vi "Draw Button Background.vi"(6 "Button Color":u32(colorbox)=11776947, 8 "error in (no error)":errorcluster, 10 "Button Size":i32=40, 11 "Button Style":T1=enum."Classic") -> (0 "error out":errorcluster={"status"=TRUE, "code"=1131, "source"="Property Node (arg 1) in Toolbar.xctl:Draw Button Background.vi<APPEND>\nProperty Name: <b>Colors [4]</b>"}, 1 "On Picture":picture, 2 "Hover Picture":picture, 3 "Off Picture":picture)   [LabVIEW 2012, in "Toolbar.xctl"]
doc: "Responsible for genertating the background image of the button. This is derived from boolean button controls of the various possible styles, each of which is then resized to the correct size and is used to generate the image of the button background."
uses:
  Toolbar.xctl
  Button_Class/Type Defs/Button Style.ctl
  Button_Class/Button.lvclass
panel:
  in  "Metallic":bool
  in  "NI Thene":bool
  in  "Silver":bool
  in  "Rounded Buttons":bool
  in  "Modern":bool
  in  "Classic":bool
  in  "System":bool
  # "Button Styles"
  # "System"
  # "Modern"
  # "Classic"
  # "Rounded"
  # "Silver"
  # "NI Theme"
  # "Metallic"
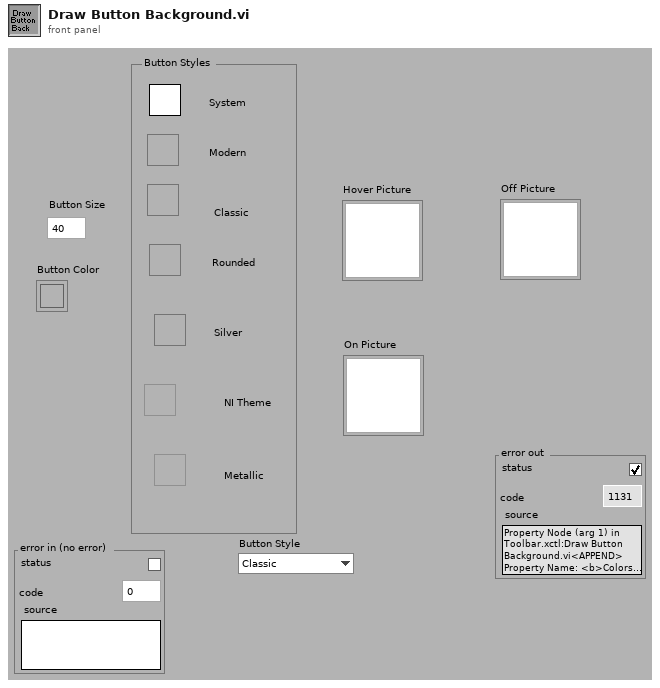
[diagram p1: front panel]
types:
  T1 = typedef "Button.lvclass/Button Style.ctl" = enum16{"System", "Modern", "Classic", "Rounded", "Silver", "Ni Theme", "Metallic"}
  T2 = cluster{"Button Color":u32, "Button Color":u32}[]
  T3 = typedef "imagedata.ctl" = cluster{"image type":i32, "image depth":i32, "image":u8[], "mask":u8[], "colors":u32[], "Rectangle":cluster{"left":i16, "top":i16, "right":i16, "bottom":i16}}
  T4 = cluster{i32, i32, "Button Size":i32, "Button Size":i32}
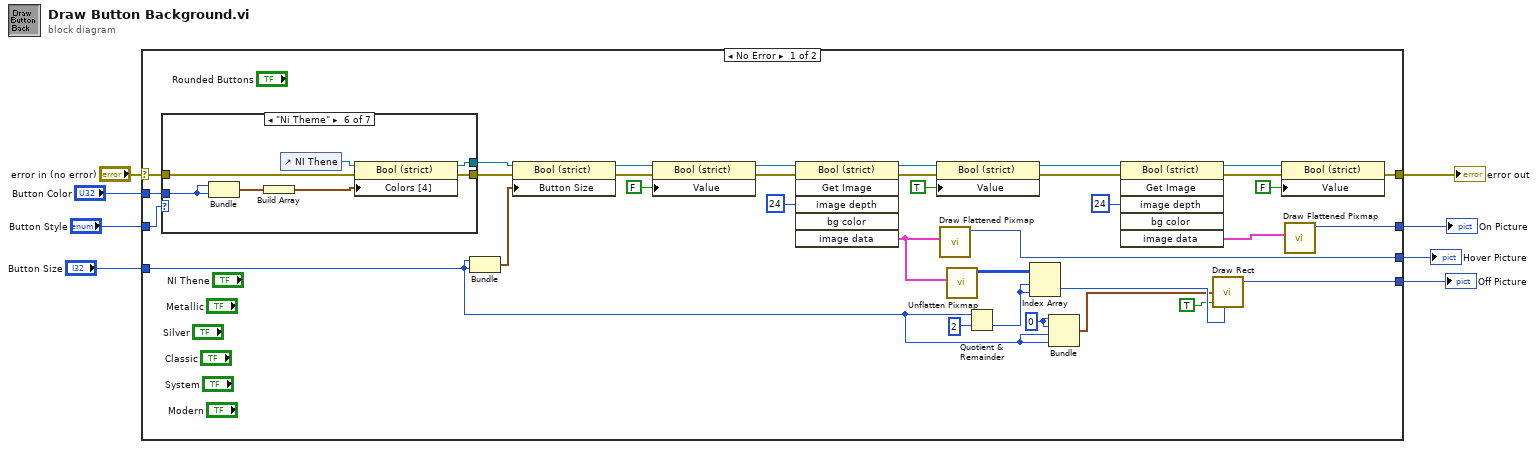
[diagram p0: block diagram]
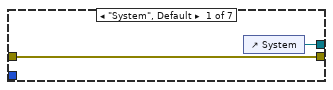
[diagram p2: hidden frame]
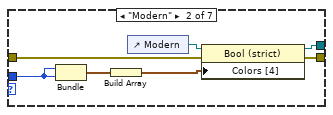
[diagram p3: hidden frame]
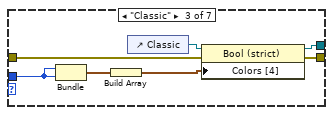
[diagram p4: hidden frame]
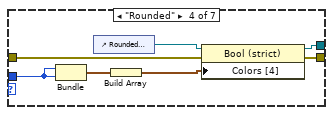
[diagram p5: hidden frame]
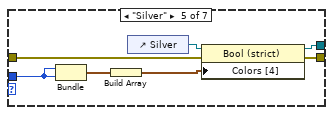
[diagram p6: hidden frame]
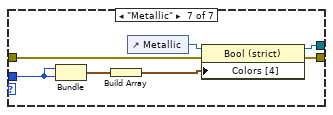
[diagram p7: hidden frame]
diagram:
  n1 = case shown="No Error" "error in (no error)" {
    selector: "error in (no error)" -> [w15 w88]
    tunnel: "Button Size" -> [w24 _]
    tunnel: [w20 w88] -> w6
    tunnel: [w23 _] -> w5
    tunnel: [w22 _] -> w4
    tunnel: [w21 _] -> w3
    tunnel: "Button Style" -> [w16 _]
    tunnel: "Button Color" -> [w11 _]
    frame No Error {
      w40 = 0
      n2 = case shown="\"Ni Theme\"" w16 {
        tunnel: w15 -> [w44 w46 w53 w61 w68 w75 w82]
        tunnel: [w45 w51 w58 w65 w72 w79 w86] -> w14
        tunnel: [w44 w52 w59 w66 w73 w80 w87] -> w13
        tunnel: w11 -> [_ w49 w57 w64 w71 w78 w85]
        frame "System", Default {
          n3 = control-ref of="System"() -> (w45:refnum<vi>)
        }
        frame "Modern" {
          n4 = Bundle("Button Color"=w49, "Button Color"=w49) -> (w48:cluster{"Button Color":u32, "Button Color":u32})  [unwired: 1 out]
          n5 = Build Array(w48) -> (w47:T2)
          n6 = control-ref of="Modern"() -> (w50:refnum<vi>)
          n7 = property class="Bool (strict)"(reference=w50, error in=w46, "Colors [4]"=w47) -> (reference out=w51:refnum<vi>, error out=w52:errorcluster)
        }
        frame "Classic" {
          n8 = Bundle("Button Color"=w57, "Button Color"=w57) -> (w56:cluster{"Button Color":u32, "Button Color":u32})  [unwired: 1 out]
          n9 = Build Array(w56) -> (w55:T2)
          n10 = control-ref of="Classic"() -> (w54:refnum<vi>)
          n11 = property class="Bool (strict)"(reference=w54, error in=w53, "Colors [4]"=w55) -> (reference out=w58:refnum<vi>, error out=w59:errorcluster)
        }
        frame "Rounded" {
          n12 = Bundle("Button Color"=w64, "Button Color"=w64) -> (w63:cluster{"Button Color":u32, "Button Color":u32})  [unwired: 1 out]
          n13 = control-ref of="Rounded Buttons"() -> (w60:refnum<vi>)
          n14 = Build Array(w63) -> (w62:T2)
          n15 = property class="Bool (strict)"(reference=w60, error in=w61, "Colors [4]"=w62) -> (reference out=w65:refnum<vi>, error out=w66:errorcluster)
        }
        frame "Silver" {
          n16 = Bundle("Button Color"=w71, "Button Color"=w71) -> (w70:cluster{"Button Color":u32, "Button Color":u32})  [unwired: 1 out]
          n17 = Build Array(w70) -> (w69:T2)
          n18 = control-ref of="Silver"() -> (w67:refnum<vi>)
          n19 = property class="Bool (strict)"(reference=w67, error in=w68, "Colors [4]"=w69) -> (reference out=w72:refnum<vi>, error out=w73:errorcluster)
        }
        frame "Ni Theme" {
          n20 = Bundle("Button Color"=w78, "Button Color"=w78) -> (w77:cluster{"Button Color":u32, "Button Color":u32})  [unwired: 1 out]
          n21 = Build Array(w77) -> (w76:T2)
          n22 = control-ref of="NI Thene"() -> (w74:refnum<vi>)
          n23 = property class="Bool (strict)"(reference=w74, error in=w75, "Colors [4]"=w76) -> (reference out=w79:refnum<vi>, error out=w80:errorcluster)
        }
        frame "Metallic" {
          n24 = Bundle("Button Color"=w85, "Button Color"=w85) -> (w84:cluster{"Button Color":u32, "Button Color":u32})  [unwired: 1 out]
          n25 = Build Array(w84) -> (w83:T2)
          n26 = control-ref of="Metallic"() -> (w81:refnum<vi>)
          n27 = property class="Bool (strict)"(reference=w81, error in=w82, "Colors [4]"=w83) -> (reference out=w86:refnum<vi>, error out=w87:errorcluster)
        }
      }
      n28 = Bundle("Button Size"=w24, "Button Size"=w24) -> (w35:cluster{"Button Size":i32, "Button Size":i32})  [unwired: 1 out]
      n29 = property on="Property Node" class="Bool (strict)"(reference=w14, error in=w13, "Button Size"=w35) -> (reference out=w18:refnum<vi>, error out=w26:errorcluster)
      n30 = property on="Property Node" class="Bool (strict)"(reference=w18, error in=w26, "Value"=FALSE ("Boolean")) -> (reference out=w17:refnum<vi>, error out=w27:errorcluster)
      n31 = invoke on="Invoke Node" class="Bool (strict)" method="Get Image"(reference=w17, error in=w27, "image depth"=24 ("Image Depth")) -> (reference out=w10:refnum<vi>, error out=w30:errorcluster, "image data"=w37:T3)  [unwired: 3 in, 3 out]
      n32 = property on="Property Node" class="Bool (strict)"(reference=w10, error in=w30, "Value"=TRUE ("Boolean")) -> (reference out=w9:refnum<vi>, error out=w28:errorcluster)
      n33 = call <vilib>:"Draw Flattened Pixmap.vi"("image data"=w37) -> ("new picture"=w21:picture)  [unwired: 1 in, 7 out]
      n34 = call <vilib>:"Unflatten Pixmap.vi"("image data"=w37) -> ("24-bit pixmap"=w38:u32[][])  [unwired: 10 out]
      n35 = Quotient & Remainder(x=w24, y=2) -> (floor(x/y)=w39:i32)  [unwired: 1 out]
      n36 = Index Array(array=w38, index (row)=w39, index (col)=w39) -> (element=w43:u32)
      n37 = Bundle(w40, w40, "Button Size"=w24, "Button Size"=w24) -> (w41:T4)  [unwired: 1 out]
      n38 = invoke on="Invoke Node" class="Bool (strict)" method="Get Image"(reference=w9, error in=w28, "image depth"=24 ("Image Depth")) -> (reference out=w19:refnum<vi>, error out=w33:errorcluster, "image data"=w32:T3)  [unwired: 3 in, 3 out]
      n39 = call <vilib>:"Draw Rect.vi"("rect"=w41, "fill?(F)"=TRUE, "color(black)"=w43) -> ("new picture"=w23:picture)  [unwired: 2 in, 4 out]
      n40 = property on="Property Node" class="Bool (strict)"(reference=w19, error in=w33, "Value"=FALSE ("Boolean")) -> (error out=w20:errorcluster)  [unwired: 1 out]
      n41 = call <vilib>:"Draw Flattened Pixmap.vi"("image data"=w32) -> ("new picture"=w22:picture)  [unwired: 1 in, 7 out]
    }
    frame Error {
    }
  }
  "Hover Picture" <- w3
  "On Picture" <- w4
  "Off Picture" <- w5
  "error out" <- w6
